vi "Write Device State Information Msg.vi"(10 "Device State Information Msg":refnum<class "Device State Information Msg.lvclass">, 11 "EMS Generic in":refnum<class "EMS Generic.lvclass">) -> (3 "EMS Generic out":refnum<class "EMS Generic.lvclass">)   [LabVIEW 2018, in "EMS Generic Actor.lvlib" / "EMS Generic.lvclass"]
uses:
  EMS Generic.lvclass
  EMS Generic Messages/Device State Information Msg/Device State Information Msg.lvclass
  EMS Generic.lvclass/EMS Generic.ctl
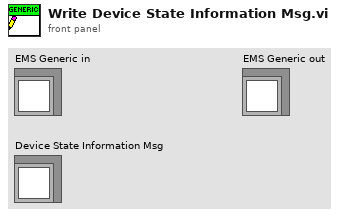
[diagram p1: front panel]
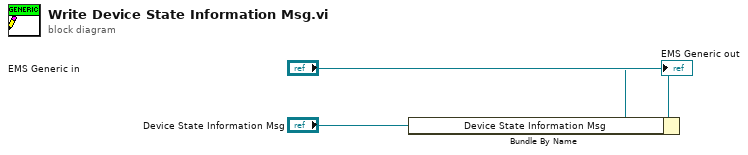
[diagram p0: block diagram]
diagram:
  n1 = Bundle By Name(cluster="EMS Generic in", "Device State Information Msg"="Device State Information Msg") -> (→"EMS Generic out":refnum<class "EMS Generic.lvclass">)
